vi "MoveMI_in_focus.vi"(8 "error in (no error)":errorcluster) -> (0 "error out":errorcluster)   [LabVIEW 2020]
panel:
  out "No errors =T":bool
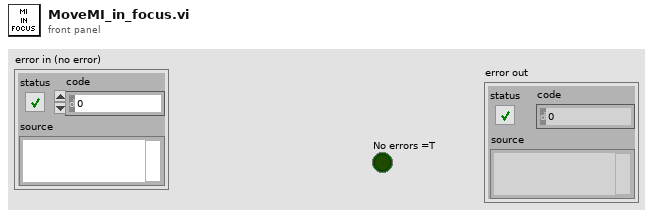
[diagram p1: front panel]
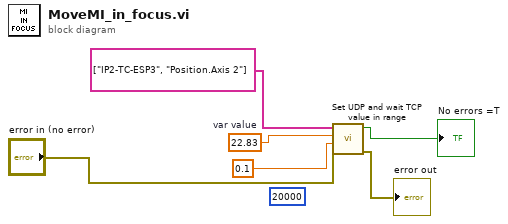
[diagram p0: block diagram]
diagram:
  (unwired) 20000 ("slow timeout ms (3000)")
  w6 = 22.83  # var value
  n1 = call "Set UDP and wait TCP value in range.vi"("error in (no error)"="error in (no error)", "tolerance"=0.1, "set value"=w6, "device and variable"=string[] ["IP2-TC-ESP3", "Position.Axis 2"] ("dev variable alias Motors X")) -> ("error out"=→"error out":errorcluster, "In range is True"=→"No errors =T":bool)  [unwired: 6 in]
